vi "Manual Drive.vi"(10 "Turn Power":dbl, 11 "Y Power":dbl) -> (2 "X Out":dbl, 3 "Y Out":dbl)   [LabVIEW 2017]
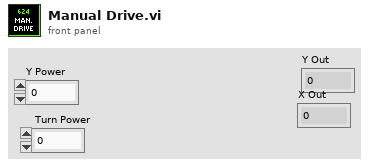
[diagram p1: front panel]
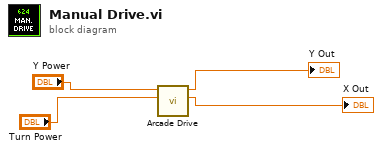
[diagram p0: block diagram]
diagram:
  n1 = call "Arcade Drive.vi"("Turn Power"="Turn Power", "Y Power"="Y Power") -> ("Right Motor Output"=→"X Out":dbl, "Left Motor Output"=→"Y Out":dbl)  [unwired: 8 in]
